vi "Get Caster Wheel Parameters.vi"(8 "error in (no error)":errorcluster, 11 "caster wheel in":refnum<class "NI_Robotics_Caster Wheel.lvclass">) -> (0 "error out":errorcluster, 2 "caster parameters":T1={"forward offset"=0.0, "caster gear ratio"=1.0}, 3 "caster wheel out":refnum<class "NI_Robotics_Caster Wheel.lvclass">)   [LabVIEW 2017, in "NI_Robotics_Caster Wheel.lvclass"]
uses:
  <vilib>/robotics/Steering/Caster Wheel/NI_Robotics_Caster Wheel.lvclass
  <vilib>/robotics/Steering/Caster Wheel/Caster Wheel Parameters.ctl
  <vilib>/robotics/Steering/Caster Wheel/NI_Robotics_Caster Wheel.lvclass/NI_Robotics_Caster Wheel.ctl
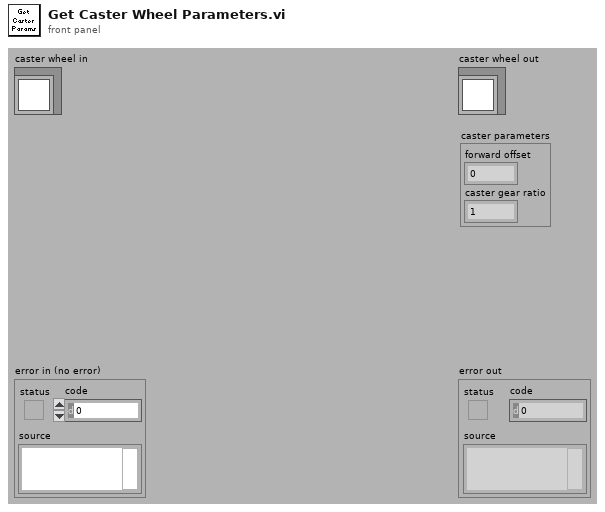
[diagram p1: front panel]
types:
  T1 = typedef "NI_Robotics_Caster Wheel.lvclass/Caster Wheel Parameters.ctl" = cluster{"forward offset":dbl, "caster gear ratio":dbl}
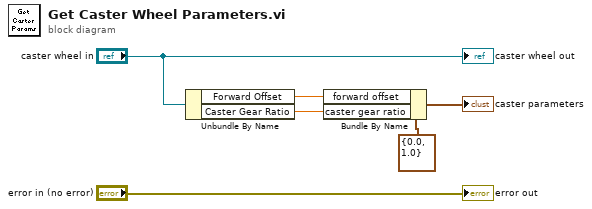
[diagram p0: block diagram]
diagram:
  n1 = Unbundle By Name("caster wheel in") -> ("Forward Offset"=w3:dbl, "Caster Gear Ratio"=w2:dbl)
  n2 = Bundle By Name(cluster=T1 {"forward offset"=0.0, "caster gear ratio"=1.0} ("caster wheel parameters"), "forward offset"=w3, "caster gear ratio"=w2) -> (→"caster parameters":T1)
  "error out" <- "error in (no error)"
  "caster wheel out" <- "caster wheel in"
